vi "Compile Initially Connected Endpoints.vi"(8 "error in":errorcluster, 9 "Compiled Connections Buffer":T1[](array[typedef]), 10 "Communication Configuration":T3, 11 "Device Ref in":T2 format="%.0x") -> (0 "error out":errorcluster, 2 "Compiled Initial Connection Indices":i32[](array[numeric]), 3 "Device Ref out":T2 format="%.0x")   [LabVIEW 2019, in "Routing and Faulting System Explorer.lvlib"]
uses:
  Routing and Faulting System Explorer.lvlib
  Shared/Communication Configuration.ctl
  <vilib>/NI VeriStand/Custom Device API/Custom Device Item Ref.ctl
  Shared/Compiled Connection.ctl
  Shared/Routing and Faulting Hardware API/Routing and Faulting Hardware API.lvlib
  Shared/Routing and Faulting Shared.lvlib
  <vilib>/NI VeriStand/Custom Device API/Custom Device API.lvlib
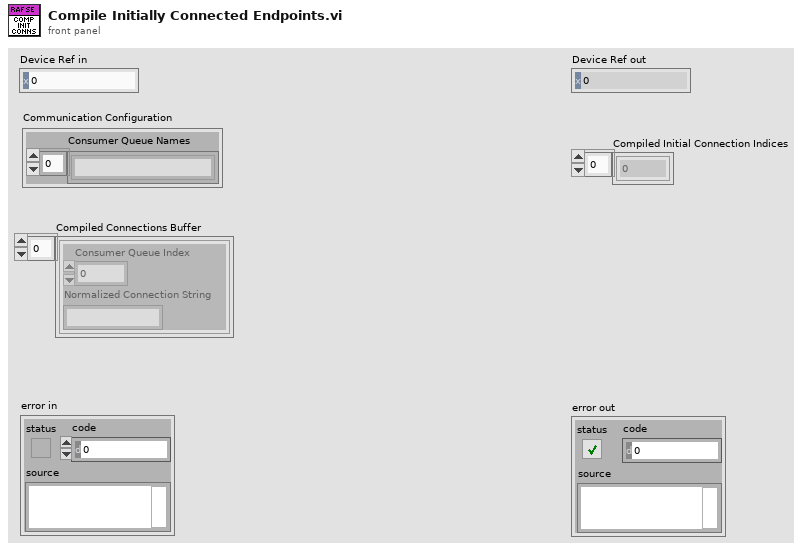
[diagram p1: front panel]
types:
  T1 = typedef "Routing and Faulting Shared.lvlib/Compiled Connection.ctl" = cluster{"Consumer Queue Index":i32, "Normalized Connection String":string}
  T2 = typedef "Custom Device API.lvlib/Custom Device Item Ref.ctl" = u64
  T3 = typedef "Routing and Faulting Shared.lvlib/Communication Configuration.ctl" = cluster{"Consumer Queue Names":string[]}
  T4 = typedef "Routing and Faulting Hardware API.lvlib/Connection.ctl" = cluster{"Endpoint 1":string, "Endpoint 2":string}
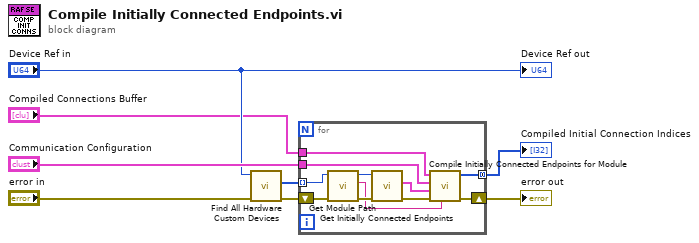
[diagram p0: block diagram]
diagram:
  n1 = call "Find All Hardware Custom Devices.vi"("error in (no error)"="error in", "Routing and Faulting Ref in"="Device Ref in") -> ("error out"=w7:errorcluster, "Hardware Refs"=w6:T2[])  [unwired: 7 in, 1 out]
  n2 = for {
    tunnel: "Compiled Connections Buffer" -> [w19]
    tunnel: "Communication Configuration" -> [w18]
    shift-right: [w17] -> w4
    shift-left: w7 -> [w13]
    tunnel: [w16] -> w3 mode=concatenating
    tunnel: w6 -> [w12] mode=indexing
    n3 = call "Get Module Path.vi"("error in (no error)"=w13, "Hardware Ref in"=w12) -> ("error out"=w10:errorcluster, "Module Path"=w9:string, "Hardware Ref out"=w11:T2)  [unwired: 6 in, 1 out]
    n4 = call "Get Initially Connected Endpoints.vi"("error in (no error)"=w10, "Hardware Ref in"=w11) -> ("error out"=w15:errorcluster, "Connections"=w14:T4[])  [unwired: 7 in, 1 out]
    n5 = call "Compile Initially Connected Endpoints for Module.vi"("Module"=w9, "error in"=w15, "Initially Connected Endpoints"=w14, "Communication Configuration"=w18, "Compiled Connections Buffer"=w19) -> ("error out"=w17:errorcluster, "Compiled Initial Connection Indices"=w16:i32[])  [unwired: 5 in]
  }
  "error out" <- w4
  "Compiled Initial Connection Indices" <- w3
  "Device Ref out" <- "Device Ref in"
